vi "Table_UI.vi"(7 "Sort by":u16(ring) items=["Packet_Number", "Timestamp", "Source", "Destination", "Protocol", "Length", "Data"], 8 "Table Control 2":refnum<vi>, 9 "Preiltered Data":string[][](array[string])=array1500x7[10500 elements], 10 "Filter String":string="Protocol == UDP AND Length > 0.7 OR Source == 192.168.1.1", 11 "Headers":string[](array[string])=["Packet Number", "Timestamp", "Source", "Destination", "Protocol", "Length", "Data"]) -> (3 "Table Control":string[][](table))   [LabVIEW 2025, in "Table_Filtering.lvlib"]
uses:
  Table_Filtering.lvlib
  c70923e2-697f-4f21-8701-1e44768d188d.vi
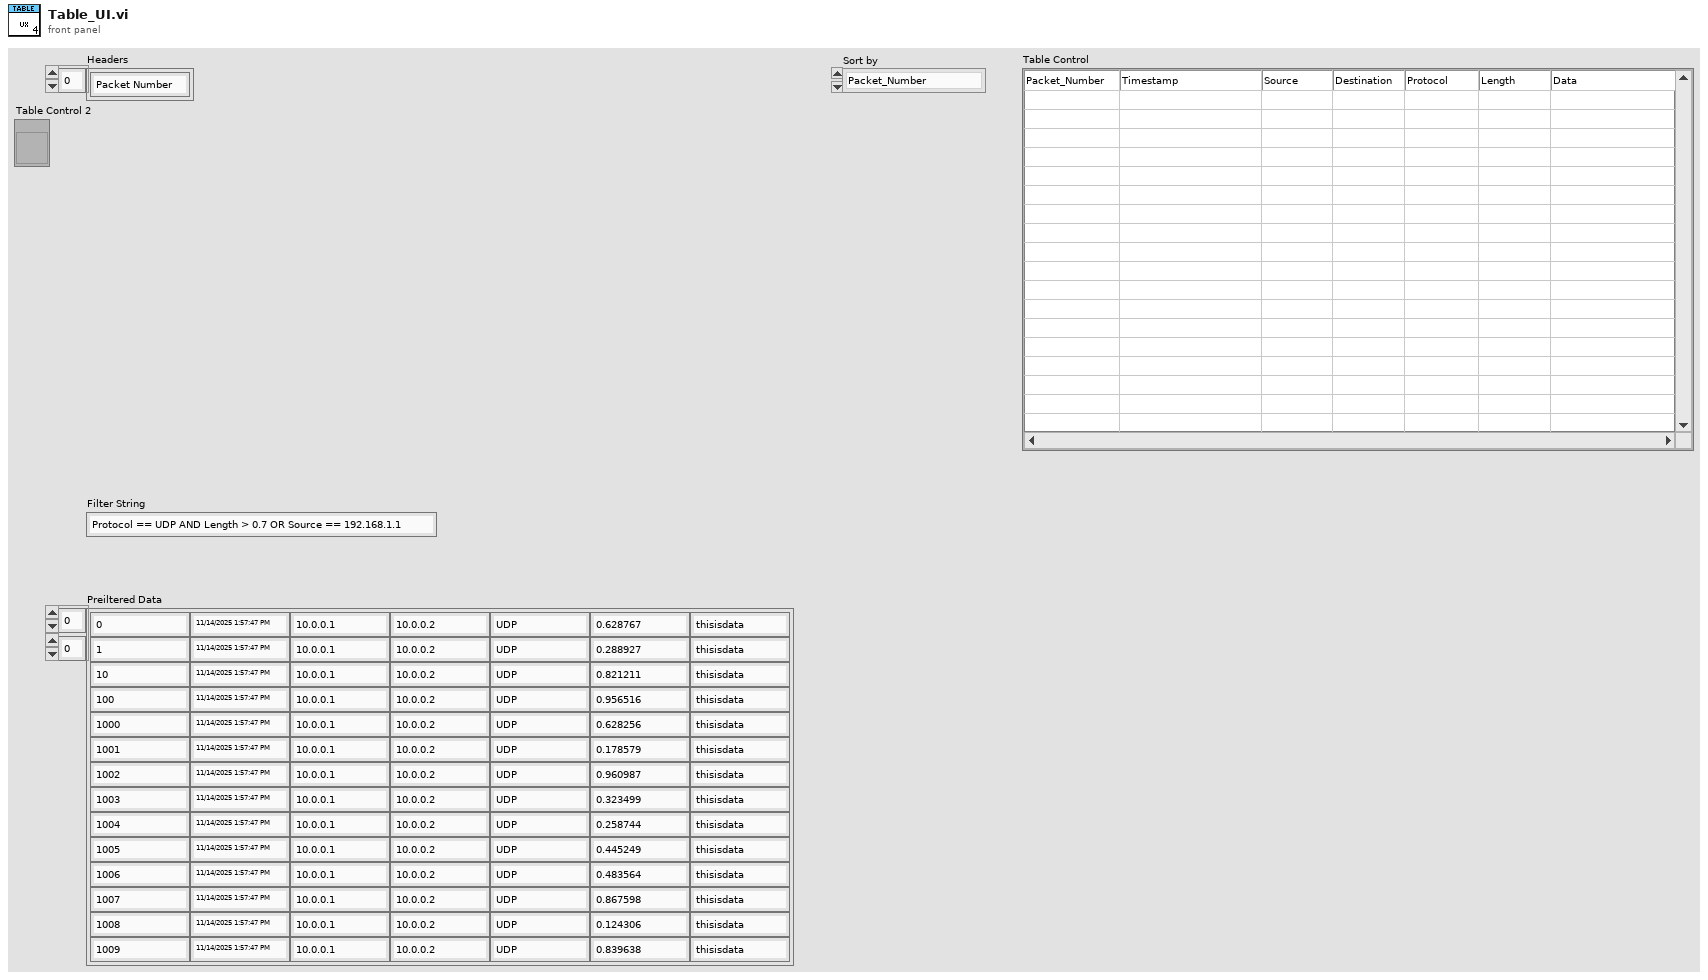
[diagram p1: front panel]
types:
  T1 = cluster{"FIELD":string, "OPERATOR":string, "VALUE":string}[]
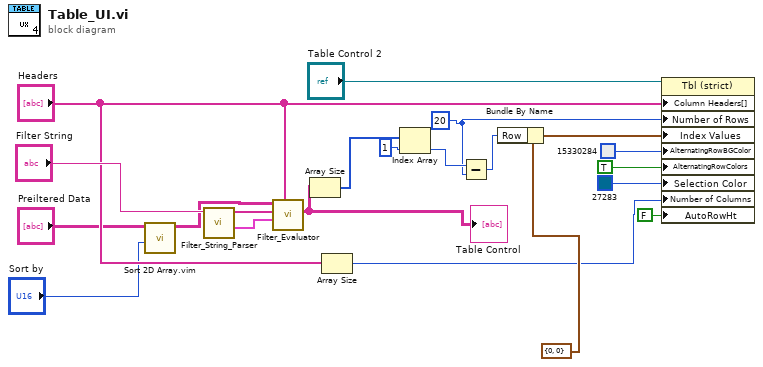
[diagram p0: block diagram]
diagram:
  w11 = 20 ("y")
  n1 = call "Sort 2D Array.vim"("index"="Sort by", "2D array"="Preiltered Data") -> ("sorted 2D array"=w4:string[][])  [unwired: 8 in, 1 out]
  n2 = call "Filter_String_Parser.vi"("Filter String"="Filter String") -> ("Comparators"=w20:T1, "Boolean Connectors"=w19:string[])  [unwired: 9 in]
  n3 = call "Filter_Evaluator.vi"("Headers"="Headers", "Comparators"=w20, "Boolean Connectors"=w19, "Prefiltered Data"=w4) -> ("Filtered Array"=w12:string[][])  [unwired: 6 in, 1 out]
  "Table Control" <- w12
  n4 = Array Size(array=w12) -> (size(s)=w18:i32[])
  n5 = Array Size(array="Headers") -> (size(s)=w9:i32)
  n6 = Index Array(array=w18, index=1) -> (element=w17:i32)
  n7 = Subtract(x=w17, y=w11) -> (x-y=w16:i32)
  n8 = Bundle By Name(cluster=cluster{"Row":u32, "Column":u32} {"Row"=0, "Column"=0} ("Index Values"), "Row"=w16) -> (w13:cluster{"Row":u32, "Column":u32})
  n9 = property on="Property Node" class="Tbl (strict)"(reference="Table Control 2", "Column Headers[]"="Headers", "Number of Rows"=w11, "Index Values"=w13, "AlternatingRowBGColor"=u32 15330284 ("Alternate Row Background Color"), "AlternatingRowColors"=TRUE ("Alternating Row Colors"), "Selection Color"=u32 27283, "Number of Columns"=w9, "AutoRowHt"=FALSE ("Autosizing Row Height")) -> ()  [unwired: 1 in, 2 out]
